vi "Create new LVLIB and add it to target item.vi"(8 "error in (no error)":errorcluster, 10 "Library path and name":path, 11 "TargetItem Ref IN":refnum<vi>) -> (0 "error out":errorcluster, 2 "Created lvlib Ref":refnum<vi>, 3 "TargetItem Ref OUT":refnum<vi>)   [LabVIEW 2015, in "NIVS_Consolidated_CDW_MetaDataObj.lvclass"]
doc: "Creates a new .lvlib and saves it on the file system. After that, add the new library to the target item in the project."
uses:
  NIVS_Consolidated_CDW_MetaDataObj.lvclass
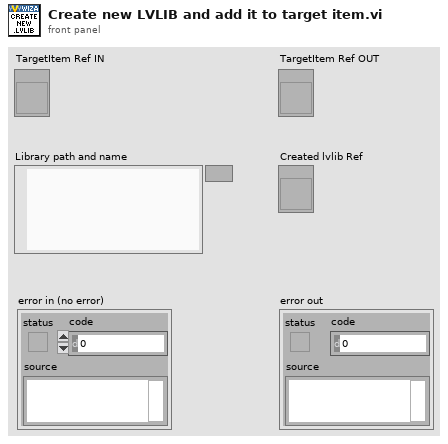
[diagram p1: front panel]
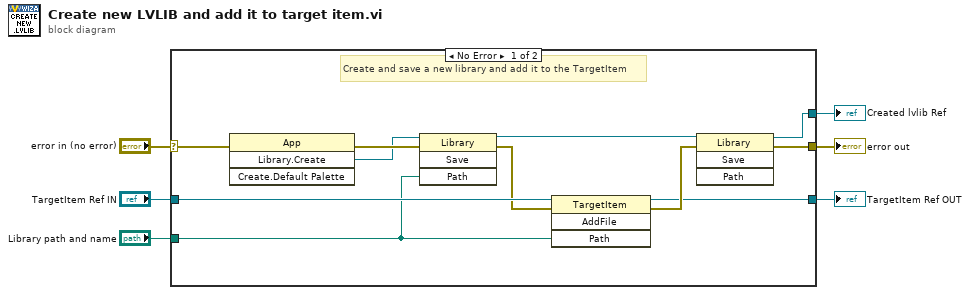
[diagram p0: block diagram]
diagram:
  n1 = case shown="No Error" "error in (no error)" {
    selector: "error in (no error)" -> [w17 w19]
    tunnel: "Library path and name" -> [w13 _]
    tunnel: [w7 _] -> w5
    tunnel: [w8 w19] -> w4
    tunnel: "TargetItem Ref IN" -> [w16 w18]
    tunnel: [w9 w18] -> w1
    frame No Error {
      # "Create and save a new library and add it to the TargetItem"
      n2 = invoke class="App" method="Library.Create"(error in=w17) -> (error out=w15:errorcluster, "Create Library"=w14:refnum<vi>)  [unwired: 3 in, 2 out]
      n3 = invoke class="Library" method="Save"(reference=w14, error in=w15, "Path"=w13) -> (reference out=w10:refnum<vi>, error out=w12:errorcluster)  [unwired: 1 in, 2 out]
      n4 = invoke class="TargetItem" method="AddFile"(reference=w16, error in=w12, "Path"=w13) -> (reference out=w9:refnum<vi>, error out=w11:errorcluster)  [unwired: 1 in, 2 out]
      n5 = invoke class="Library" method="Save"(reference=w10, error in=w11) -> (reference out=w7:refnum<vi>, error out=w8:errorcluster)  [unwired: 2 in, 2 out]
    }
    frame Error {
      # "Output default values."
    }
  }
  "Created lvlib Ref" <- w5
  "error out" <- w4
  "TargetItem Ref OUT" <- w1
